vi "Place radio button and distrubute elements.vi"(8 "error in":errorcluster, 9 "Bottom of last control":u32, 11 "radio button reference":refnum<vi>) -> (0 "error out":errorcluster, 3 "radio button reference out":refnum<vi>)   [LabVIEW 2020, in "verticalDistribution.lvlib"]
uses:
  <vilib>/Utility/vertDist/verticalDistribution.lvlib
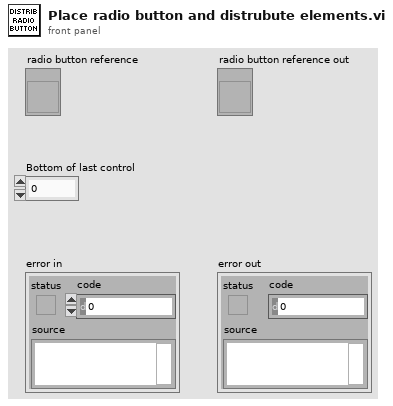
[diagram p1: front panel]
types:
  T1 = typedef "LVRectTypeDef.ctl" = cluster{"Left":i16, "Top":i16, "Right":i16, "Bottom":i16}
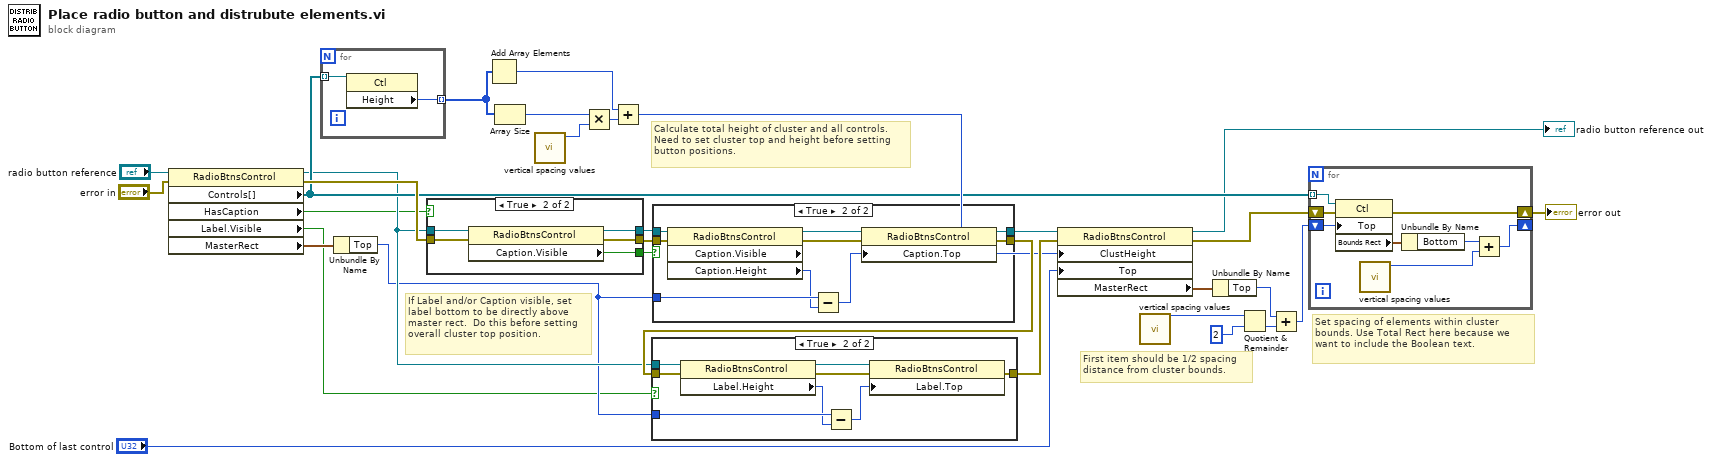
[diagram p0: block diagram]
diagram:
  # "Set spacing of elements within cluster bounds. Use Total Rect here because we want to include the Boolean text."
  # "First item should be 1/2 spacing\ndistance from cluster bounds."
  # "If Label and/or Caption visible, set \nlabel bottom to be directly above \nmaster rect.  Do this before setting\noverall cluster top position."
  # "Calculate total height of cluster and all controls.\nNeed to set cluster top and height before setting\nbutton positions."
  n1 = property class="RadioBtnsControl"(reference="radio button reference", error in="error in") -> (reference out=w17:refnum<vi>, error out=w26:errorcluster, "Controls[]"=w22:refnum<vi>[], "HasCaption"=w5:bool, "Label.Visible"=w10:bool, "MasterRect"=w12:T1)
  n2 = for {
    tunnel: w22 -> [w32] mode=indexing
    tunnel: [w33] -> w6 mode=indexing
    n3 = property class="Ctl"(reference=w32) -> ("Height"=w33:u32)  [unwired: 1 in, 2 out]
  }
  n4 = Unbundle By Name(w12) -> ("Top"=w15:i16)
  n5 = case shown="True" w5 {
    tunnel: w17 -> [w34 w38]
    tunnel: [w34 w37] -> w13
    tunnel: w26 -> [w35 w40]
    tunnel: [w35 w39] -> w27
    tunnel: [_ w36] -> w14
    frame False {
    }
    frame True {
      n6 = property class="RadioBtnsControl"(reference=w38, error in=w40) -> (reference out=w37:refnum<vi>, error out=w39:errorcluster, "Caption.Visible"=w36:bool)
    }
  }
  n7 = Add Array Elements(numeric array=w6) -> (sum=w8:u32)
  n8 = Array Size(array=w6) -> (size(s)=w9:i32)
  n9 = call <vilib>:"vertical spacing values.vi"() -> ("Control spacing"=w4:u32)  [unwired: 3 out]
  n10 = Multiply(x=w9, y=w4) -> (x*y=w7:u32)
  n11 = Add(x=w8, y=w7) -> (x+y=w24:u32)
  n12 = case shown="True" w14 {
    tunnel: w13 -> [w41 w48]
    tunnel: [w41 w46] -> w16
    tunnel: w27 -> [w42 w51]
    tunnel: [w42 w49] -> w29
    tunnel: w15 -> [_ w44]
    frame False {
    }
    frame True {
      n13 = property class="RadioBtnsControl" props=["Caption", "Visible", "Caption", "Height"](reference=w48, error in=w51) -> (reference out=w47:refnum<vi>, error out=w50:errorcluster, "Caption.Height"=w43:u32)  [unwired: 1 out]
      n14 = Subtract(x=w44, y=w43) -> (x-y=w45:u32)
      n15 = property class="RadioBtnsControl"(reference=w47, error in=w50, "Caption.Top"=w45) -> (reference out=w46:refnum<vi>, error out=w49:errorcluster)
    }
  }
  n16 = case shown="True" w10 {
    tunnel: w17 -> [_ w57]
    tunnel: w29 -> [w52 w58]
    tunnel: [w52 w60] -> w30
    tunnel: w15 -> [_ w54]
    frame False {
    }
    frame True {
      n17 = property class="RadioBtnsControl"(reference=w57, error in=w58) -> (reference out=w56:refnum<vi>, error out=w59:errorcluster, "Label.Height"=w53:u32)
      n18 = Subtract(x=w54, y=w53) -> (x-y=w55:u32)
      n19 = property class="RadioBtnsControl"(reference=w56, error in=w59, "Label.Top"=w55) -> (error out=w60:errorcluster)  [unwired: 1 out]
    }
  }
  n20 = property class="RadioBtnsControl"(reference=w16, error in=w30, "ClustHeight"=w24, "Top"="Bottom of last control") -> (reference out=→"radio button reference out":refnum<vi>, error out=w28:errorcluster, "MasterRect"=w21:T1)
  n21 = call <vilib>:"vertical spacing values.vi"() -> ("Control spacing"=w3:u32)  [unwired: 3 out]
  n22 = Unbundle By Name(w21) -> ("Top"=w20:i16)
  n23 = Quotient & Remainder(x=w3, y=u32 2) -> (floor(x/y)=w18:u32)  [unwired: 1 out]
  n24 = Add(x=w20, y=w18) -> (x+y=w11:u32)
  n25 = for {
    tunnel: w22 -> [w66] mode=indexing
    shift-right: [w62] -> _
    shift-left: w11 -> [w64]
    shift-right: [w68] -> w31
    shift-left: w28 -> [w67]
    n26 = property class="Ctl"(reference=w66, error in=w67, "Top"=w64) -> (error out=w68:errorcluster, "Bounds Rect"=w65:T1)  [unwired: 1 out]
    n27 = call <vilib>:"vertical spacing values.vi"() -> ("Control spacing"=w61:u32)  [unwired: 3 out]
    n28 = Unbundle By Name(w65) -> ("Bottom"=w63:i16)
    n29 = Add(x=w63, y=w61) -> (x+y=w62:u32)
  }
  "error out" <- w31
